vi "Move Check.vi"(6 "Round":i32, 8 "Assumed Dir":T1, 9 "Idx":i32, 10 "SpawnDist":i32, 11 "Board":refnum<data-value>) -> (0 "Direction":T1, 1 "Spawn Can End?":bool, 2 "SpawnDist out":i32)   [LabVIEW 2015, in "Formation.lvclass"]
uses:
  Formation.lvclass
  Board Cluster.ctl
  Type Defs/Direction Enum.ctl
  Type Defs/SB Type Defs.lvlib
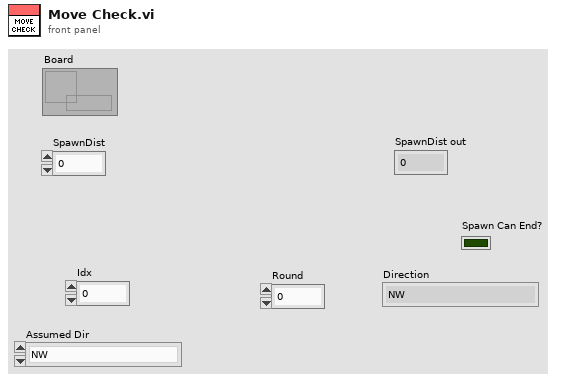
[diagram p1: front panel]
types:
  T1 = typedef "SB Type Defs.lvlib/Direction Enum.ctl" = enum16{"NW", "N", "NE", "E", "SE", "S", "SW", "W"}
  T2 = typedef "Formation.lvclass/Board Cluster.ctl" = cluster{"Board S":i32, "Pos[Idx]":cluster{"X":i32, "Y":i32}[], "Round[Idx]":i32[]}
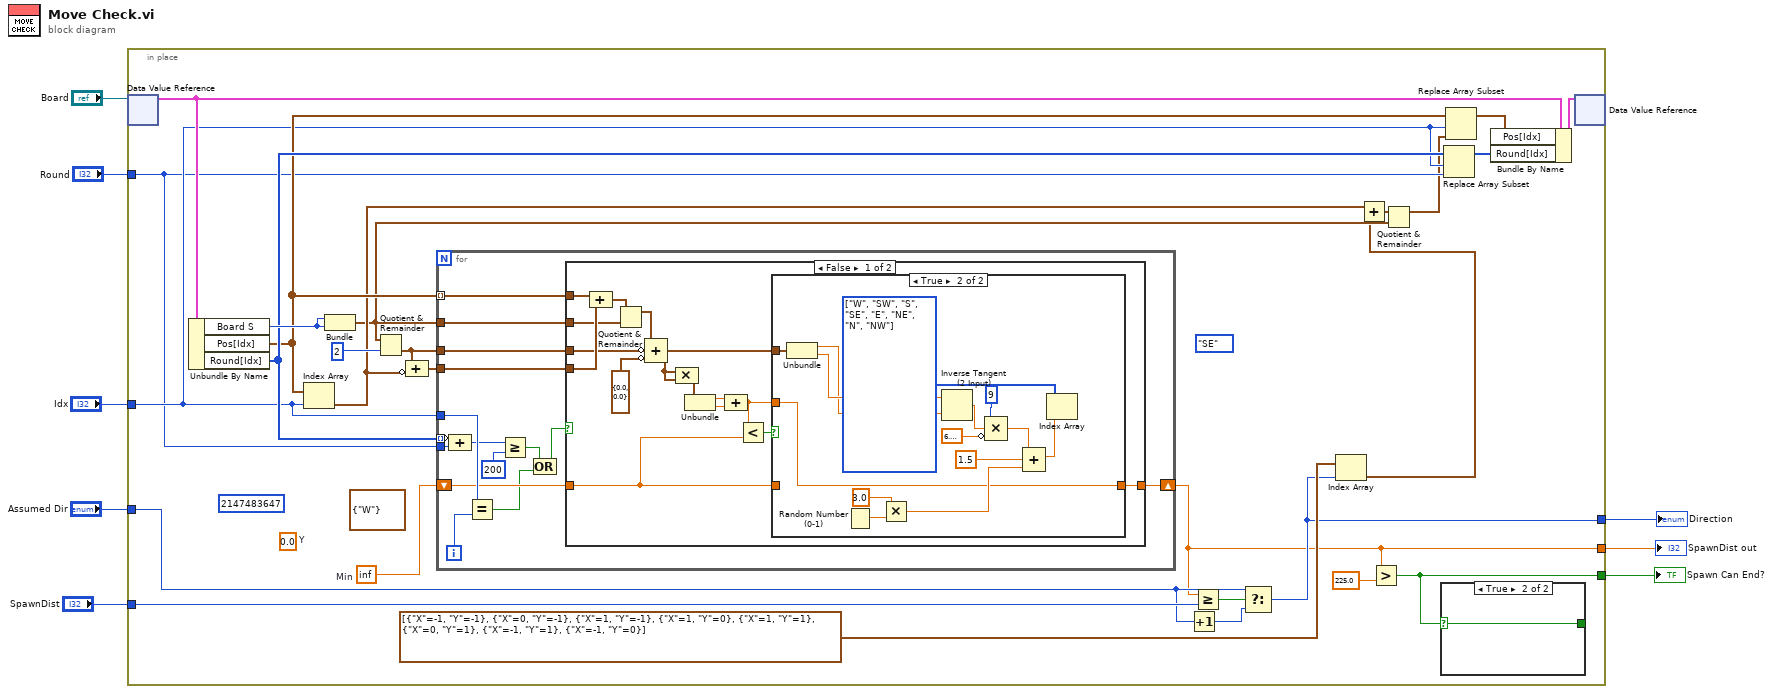
[diagram p0: block diagram]
diagram:
  n1 = in-place {
    in-place-border: "Idx" -> [w25]
    in-place-border: [w12] -> w6
    in-place-border: [w16] -> w5
    in-place-border: "Round" -> [w24]
    in-place-border: "Assumed Dir" -> [w11]
    in-place-border: "SpawnDist" -> [w14]
    in-place-border: [w9] -> w1
    w15 = inf  # Min
    (unwired) Direction_Enum."SE" ("Direction")
    (unwired) 0.0  # Y
    (unwired) cluster{"Direction":T1} {"Direction"=enum."W"}
    (unwired) 2147483647
    n2 = in-place-dvr #1("Board") -> (w29:T2)  [unwired: 1 out]
    n3 = Unbundle By Name(w29) -> ("Board S"=w35:i32, "Pos[Idx]"=w30:cluster{"X":i32, "Y":i32}[], "Round[Idx]"=w31:i32[])
    n4 = Index Array(array=w30, index=w25) -> (element=w23:cluster{"X":i32, "Y":i32})
    n5 = Bundle("Board S"=w35, "Board S"=w35) -> (w21:cluster{"Board S":i32, "Board S":i32})  [unwired: 1 in]
    n6 = Quotient & Remainder(x=w21, y=2) -> (floor(x/y)=w32:cluster{"Board S":i32, "Board S":i32})  [unwired: 1 out]
    n7 = Compound Arithmetic op=ADD(w32, invert w23) -> (w33:cluster{i32, i32})
    n8 = for {
      shift-right: [w46] -> w9
      shift-left: w15 -> [w45]
      tunnel: w33 -> [w50]
      tunnel: w30 -> [w51] mode=indexing
      tunnel: w31 -> [w41] mode=indexing
      tunnel: w25 -> [w48]
      tunnel: w32 -> [w47]
      tunnel: w21 -> [w42]
      tunnel: w24 -> [w40]
      i -> [w49]
      n9 = Compound Arithmetic op=ADD(invert w41, w40) -> (w39:i32)
      n10 = Equal?(x=w48, y=w49) -> (x = y?=w44:bool)
      n11 = Greater Or Equal?(x=w39, y=200) -> (x >= y?=w37:bool)
      n12 = Compound Arithmetic op=OR(w37, w44) -> (w43:bool)
      n13 = case shown="False" w43 {
        tunnel: w51 -> [w66 _]
        tunnel: w50 -> [w65 _]
        tunnel: w47 -> [w64 _]
        tunnel: [w55 w82] -> w46
        tunnel: w45 -> [w52 w82]
        tunnel: w42 -> [w62 _]
        frame False {
          n14 = Compound Arithmetic op=ADD(w66, w65) -> (w63:cluster{i32, i32})
          n15 = Quotient & Remainder(x=w63, y=w62) -> (x-y*floor(x/y)=w61:cluster{i32, i32})  [unwired: 1 out]
          n16 = Compound Arithmetic op=unknown(w61, invert w64, invert cluster{"Board S":dbl, "Board S":dbl} {"Board S"=0.0, "Board S"=0.0} ("value")) -> (w54:cluster{dbl, dbl})
          n17 = Compound Arithmetic op=MULTIPLY(w54, w54) -> (w58:cluster{dbl, dbl})
          n18 = Unbundle(w58) -> (w59:dbl, w60:dbl)
          n19 = Compound Arithmetic op=ADD(w59, w60) -> (w53:dbl)
          n20 = Less?(x=w53, y=w52) -> (x < y?=w56:bool)
          n21 = case shown="True" w56 {
            tunnel: w52 -> [w67 _]
            tunnel: [w67 w68] -> w55
            tunnel: w54 -> [_ w74]
            tunnel: w53 -> [_ w68]
            frame False {
            }
            frame True {
              w75 = T1[] [enum."W", enum."SW", enum."S", enum."SE", enum."E", enum."NE", enum."N", enum."NW"] items=["NW", "N", "NE", "E", "SE", "S", "SW", "W"]
              n22 = Unbundle(w74) -> (w72:dbl, w73:dbl)
              n23 = Random Number (0-1)() -> (number: 0 to 1=w71:dbl)
              n24 = Multiply(x=3.0, y=w71) -> (x*y=w69:dbl)
              n25 = Inverse Tangent (2 Input)(1:w72, 2:w73) -> (0:w79:dbl)
              n26 = Compound Arithmetic op=MULTIPLY(9, w79, invert 6.283185307179586) -> (w76:dbl)
              n27 = Compound Arithmetic op=ADD(w76, 1.5, w69) -> (w81:dbl)
              n28 = Index Array(array=w75, index=w81) -> ()  [unwired: 1 out]
            }
          }
        }
        frame True {
        }
      }
    }
    n29 = Increment(x=w11) -> (x+1=w10:T1)
    n30 = Greater Or Equal?(x=w9, y=w14) -> (x >= y?=w13:bool)
    n31 = Select(t=w11, s=w13, f=w10) -> (s? t:f=w12:T1)
    n32 = Index Array(array=cluster{"X":i32, "Y":i32}[] [{"X"=-1, "Y"=-1}, {"X"=0, "Y"=-1}, {"X"=1, "Y"=-1}, {"X"=1, "Y"=0}, {"X"=1, "Y"=1}, {"X"=0, "Y"=1}, {"X"=-1, "Y"=1}, {"X"=-1, "Y"=0}], index=w12) -> (element=w19:cluster{"X":i32, "Y":i32})
    n33 = Add(x=w23, y=w19) -> (x+y=w22:cluster{"X":i32, "Y":i32})
    n34 = Greater?(x=w9, y=225.0) -> (0:w16:bool)
    n35 = Quotient & Remainder(x=w22, y=w21) -> (x-y*floor(x/y)=w18:cluster{i32, i32})  [unwired: 1 out]
    n36 = case shown="True" w16 {
      selector: w16 -> [_ w36]
      tunnel: [_ w36] -> _
      frame False {
      }
      frame True {
      }
    }
    n37 = Replace Array Subset(array=w31, new element=w24, index=w25) -> (w26:i32[])
    n38 = Replace Array Subset(array=w30, new element=w18, index=w25) -> (w27:cluster{"X":i32, "Y":i32}[])
    n39 = Bundle By Name(cluster=w29, "Pos[Idx]"=w27, "Round[Idx]"=w26) -> (w28:T2)
    n40 = in-place-dvr #1(w28) -> ()  [unwired: 2 out]
  }
  "Direction" <- w6
  "Spawn Can End?" <- w5
  "SpawnDist out" <- w1
